vi "CaliperEntryFilter.vi"(11 "CaliperEntryList":T6[](array[typedef]) {"CaliperType" items=["Distance", "Mid Point", "Perpendicular Projection", "Lines Intersection", "Angle from Horizontal", "Angle from Vertical", "Angle Defined by 3 Points", "Angle Defined by 4 Points", "Bissecting Line", "Mid Line", "Center of Mass", "Area", "Line Fit", "Circle Fit", "Ellipse Fit"]}) -> (3 "FilteredCaliperEntry":T1[](array[typedef]) {"CaliperType" items=["Distance", "Mid Point", "Perpendicular Projection", "Lines Intersection", "Angle from Horizontal", "Angle from Vertical", "Angle Defined by 3 Points", "Angle Defined by 4 Points", "Bissecting Line", "Mid Line", "Center of Mass", "Area", "Line Fit", "Circle Fit", "Ellipse Fit"]})   [LabVIEW 2019]
uses:
  Controls/CaliperDataEntry.ctl
  Controls/CaliperType.ctl
  Controls/SelectionListEntry.ctl
  Controls/SelectionListEntryPointType.ctl
  Controls/CaliperResult.ctl
  Controls/CaliperDataEntry_SinglePoint.ctl
  Controls/CaliperResult_SinglePoint.ctl
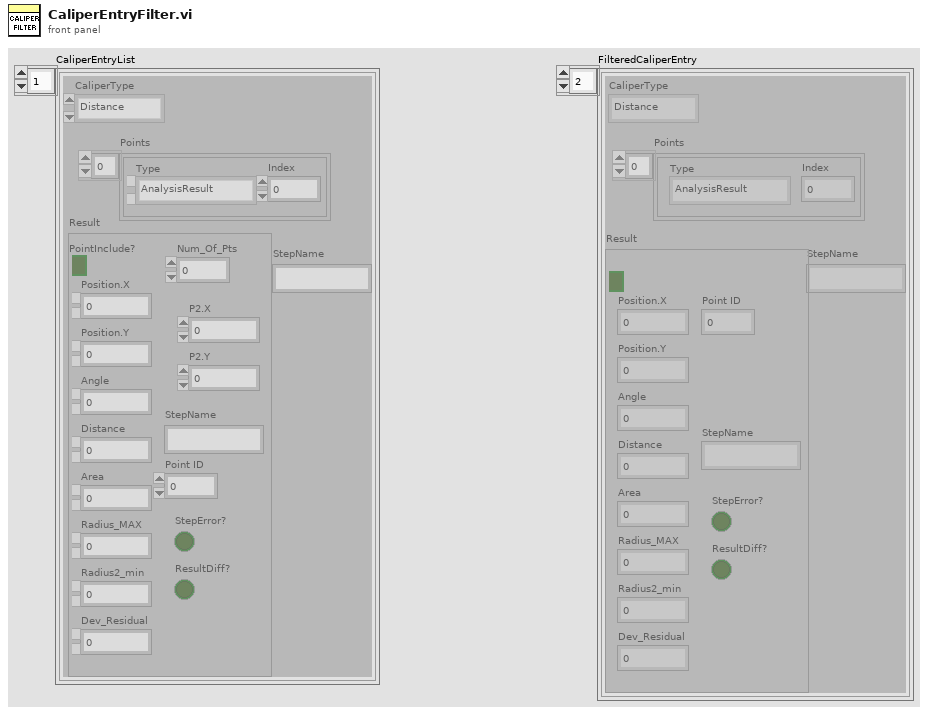
[diagram p1: front panel]
types:
  T1 = typedef "CaliperDataEntry_SinglePoint.ctl" = cluster{"CaliperType":T2, "Points":T3[], "Result":T5, "StepName":string}
  T2 = typedef "CaliperType.ctl" = u32
  T3 = typedef "SelectionListEntry.ctl" = cluster{"Type":T4, "Index":i32}
  T4 = typedef "SelectionListEntryPointType.ctl" = enum16{"AnalysisResult", "CaliperResult"}
  T5 = typedef "CaliperResult_SinglePoint.ctl" = cluster{"PointInclude?":bool, "Position.X":dbl, "Position.Y":dbl, "Angle":dbl, "Distance":dbl, "Area":dbl, "Radius_MAX":dbl, "Radius2_min":dbl, "Dev_Residual":dbl, "StepName":string, "Point ID":u8, "StepError?":bool, "ResultDiff?":bool}
  T6 = typedef "CaliperDataEntry.ctl" = cluster{"CaliperType":T2, "Points":T3[], "Result":T7, "StepName":string}
  T7 = typedef "CaliperResult.ctl" = cluster{"PointInclude?":bool, "Num_Of_Pts":u8, "Position.X":dbl, "Position.Y":dbl, "Angle":dbl, "Distance":dbl, "Area":dbl, "Radius_MAX":dbl, "Radius2_min":dbl, "Dev_Residual":dbl, "P2.X":dbl, "P2.Y":dbl, "StepName":string, "Point ID":u8, "StepError?":bool, "ResultDiff?":bool}
  T8 = cluster{"PointInclude?":bool, "Position.X":dbl, "Position.Y":dbl, "Angle":dbl, "Distance":dbl, "Area":dbl, "Radius_MAX":dbl, "Radius2_min":dbl, "Dev_Residual":dbl, "StepName":string, "Point ID":u8, "StepError?":bool, "ResultDiff?":bool}
  T9 = cluster{"PointInclude?":bool, "P2.X":dbl, "P2.Y":dbl, "Angle":dbl, "Distance":dbl, "Area":dbl, "Radius_MAX":dbl, "Radius2_min":dbl, "Dev_Residual":dbl, "StepName":string, "Point ID":u8, "StepError?":bool, "ResultDiff?":bool}
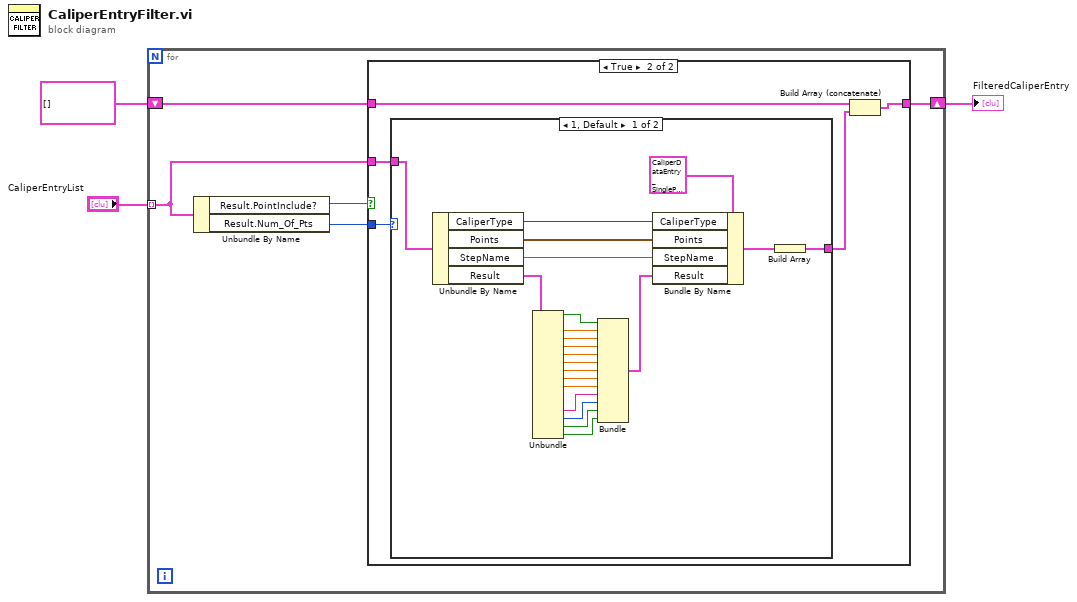
[diagram p0: block diagram]
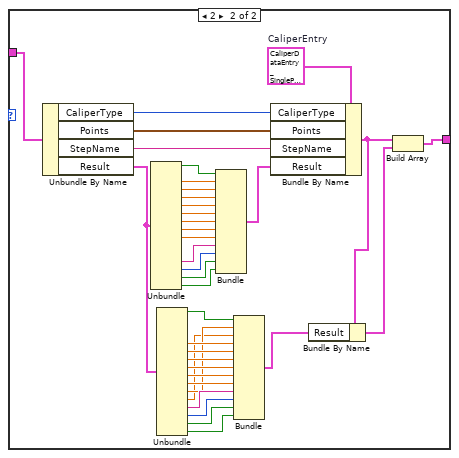
[diagram p3: hidden frame]
diagram:
  n1 = for {
    tunnel: "CaliperEntryList" -> [w7] mode=indexing
    shift-right: [w5] -> w1
    shift-left: T1[] [] ("Array") -> [w6]
    n2 = Unbundle By Name(w7) -> ("Result.PointInclude?"=w8:bool, "Result.Num_Of_Pts"=w4:u8)
    n3 = case shown="True" w8 {
      tunnel: w7 -> [_ w11]
      tunnel: w6 -> [w9 w14]
      tunnel: [w9 w13] -> w5
      tunnel: w4 -> [_ w12]
      frame False {
      }
      frame True {
        n4 = case shown="1, Default" w12 {
          tunnel: w11 -> [w36 w73]
          tunnel: [w30 w68] -> w10
          frame 1, Default {
            n5 = Unbundle By Name(w36) -> ("CaliperType"=w34:T2, "Points"=w33:T3[], "StepName"=w32:string, "Result"=w29:T7)
            n6 = Unbundle(w29) -> ("PointInclude?"=w28:bool, "Position.X"=w27:dbl, "Position.Y"=w26:dbl, "Angle"=w25:dbl, "Distance"=w24:dbl, "Area"=w23:dbl, "Radius_MAX"=w22:dbl, "Radius2_min"=w21:dbl, "Dev_Residual"=w20:dbl, "StepName"=w19:string, "Point ID"=w18:u8, "StepError?"=w16:bool, "ResultDiff?"=w15:bool)  [unwired: 3 out]
            n7 = Bundle("PointInclude?"=w28, "Position.X"=w27, "Position.Y"=w26, "Angle"=w25, "Distance"=w24, "Area"=w23, "Radius_MAX"=w22, "Radius2_min"=w21, "Dev_Residual"=w20, "StepName"=w19, "Point ID"=w18, "StepError?"=w16, "ResultDiff?"=w15) -> (w17:T8)  [unwired: 1 in]
            n8 = Bundle By Name(cluster=T1 {"CaliperType"=0, "Points"=[], "Result"={"PointInclude?"=FALSE, "Position.X"=0.0, "Position.Y"=0.0, "Angle"=0.0, "Distance"=0.0, "Area"=0.0, "Radius_MAX"=0.0, "Radius2_min"=0.0, "Dev_Residual"=0.0, "StepName"="", "Point ID"=0, "StepError?"=FALSE, "ResultDiff?"=FALSE}, "StepName"=""} ("CaliperEntry"), "CaliperType"=w34, "Points"=w33, "StepName"=w32, "Result"=w17) -> (w31:T1)
            n9 = Build Array(w31) -> (w30:T1[])
          }
          frame 2 {
            w72 = T1 {"CaliperType"=0, "Points"=[], "Result"={"PointInclude?"=FALSE, "Position.X"=0.0, "Position.Y"=0.0, "Angle"=0.0, "Distance"=0.0, "Area"=0.0, "Radius_MAX"=0.0, "Radius2_min"=0.0, "Dev_Residual"=0.0, "StepName"="", "Point ID"=0, "StepError?"=FALSE, "ResultDiff?"=FALSE}, "StepName"=""}  # CaliperEntry
            n10 = Unbundle By Name(w73) -> ("CaliperType"=w71:T2, "Points"=w70:T3[], "StepName"=w69:string, "Result"=w44:T7)
            n11 = Unbundle(w44) -> ("PointInclude?"=w67:bool, "Position.X"=w66:dbl, "Position.Y"=w65:dbl, "Angle"=w64:dbl, "Distance"=w63:dbl, "Area"=w62:dbl, "Radius_MAX"=w61:dbl, "Radius2_min"=w60:dbl, "Dev_Residual"=w59:dbl, "StepName"=w58:string, "Point ID"=w57:u8, "StepError?"=w40:bool, "ResultDiff?"=w38:bool)  [unwired: 3 out]
            n12 = Unbundle(w44) -> ("PointInclude?"=w47:bool, "Angle"=w48:dbl, "Distance"=w49:dbl, "Area"=w50:dbl, "Radius_MAX"=w51:dbl, "Radius2_min"=w52:dbl, "Dev_Residual"=w53:dbl, "P2.X"=w43:dbl, "P2.Y"=w42:dbl, "StepName"=w54:string, "Point ID"=w55:u8, "StepError?"=w39:bool, "ResultDiff?"=w37:bool)  [unwired: 3 out]
            n13 = Bundle("PointInclude?"=w67, "Position.X"=w66, "Position.Y"=w65, "Angle"=w64, "Distance"=w63, "Area"=w62, "Radius_MAX"=w61, "Radius2_min"=w60, "Dev_Residual"=w59, "StepName"=w58, "Point ID"=w57, "StepError?"=w40, "ResultDiff?"=w38) -> (w56:T8)  [unwired: 1 in]
            n14 = Bundle("PointInclude?"=w47, "P2.X"=w43, "P2.Y"=w42, "Angle"=w48, "Distance"=w49, "Area"=w50, "Radius_MAX"=w51, "Radius2_min"=w52, "Dev_Residual"=w53, "StepName"=w54, "Point ID"=w55, "StepError?"=w39, "ResultDiff?"=w37) -> (w41:T9)  [unwired: 1 in]
            n15 = Bundle By Name(cluster=w72, "CaliperType"=w71, "Points"=w70, "StepName"=w69, "Result"=w56) -> (w46:T1)
            n16 = Bundle By Name(cluster=w46, "Result"=w41) -> (w45:T1)
            n17 = Build Array(w46, w45) -> (w68:T1[])
          }
        }
        n18 = Build Array (concatenate)(w14, w10) -> (w13:T1[])
      }
    }
  }
  "FilteredCaliperEntry" <- w1
